vi "Example.vi"() -> ()   [LabVIEW 2024]
uses:
  Users/crogers/GitHub/ME121-25/LabVIEW/SerialVIs/subs/portX.xctl
panel:
  in  "CtrlC":bool
  in  "Send Code":bool
  in  "Code to run":string="import time\n\nfor i in range(10):\n    print(i)\n    time.sleep(1)\n"
  in  "portX":refnum<visa-resource-name>(xcontrol)
  in  "Send it":bool
  in  "Stop Button":bool
  in  "Single line":string="2+2"
  out "reply":string
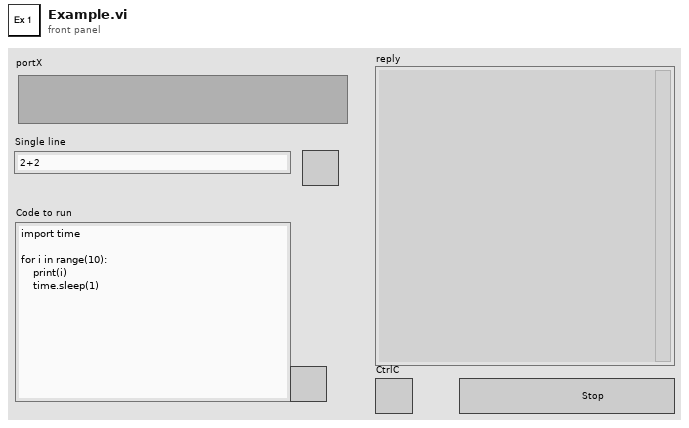
[diagram p1: front panel]
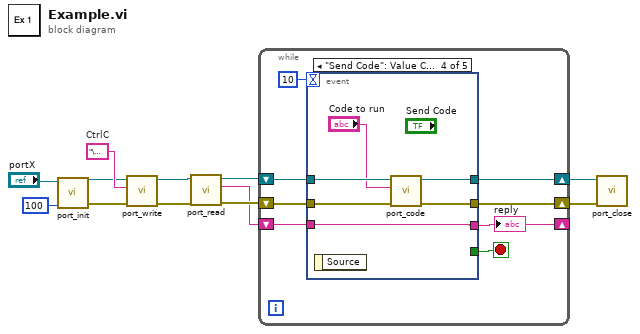
[diagram p0: block diagram]
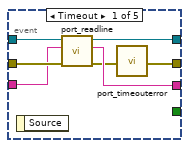
[diagram p2: hidden frame]
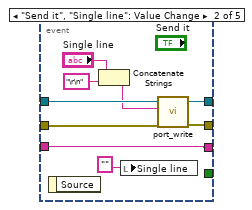
[diagram p3: hidden frame]
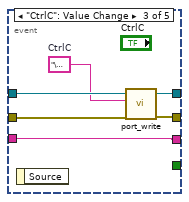
[diagram p4: hidden frame]
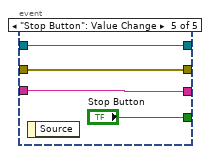
[diagram p5: hidden frame]
diagram:
  w12 = "\u0003"  # CtrlC
  n1 = call <userlib>:"port_init.vi"("Timeout (ms)"=u32 100, "VISA Refnum in"="portX") -> ("error out"=w10:errorcluster, "VISA Refnum out"=w11:refnum<visa-resource-name>)  [unwired: 8 in]
  n2 = call <userlib>:"port_write.vi"("error in (no error)"=w10, "write buffer"=w12, "VISA Refnum in"=w11) -> ("error out"=w6:errorcluster, "VISA Refnum out"=w7:refnum<visa-resource-name>)  [unwired: 7 in]
  n3 = call <userlib>:"port_read.vi"("error in (no error)"=w6, "VISA Refnum in"=w7) -> ("error out"=w5:errorcluster, "reply"=w3:string, "VISA Refnum out"=w4:refnum<visa-resource-name>)  [unwired: 7 in]
  n4 = while {
    shift-right: [w17] -> w8
    shift-left: w4 -> [w20]
    shift-right: [w18] -> w9
    shift-left: w5 -> [w19]
    shift-right: [w14] -> _
    shift-left: w3 -> [w13]
    stop <- w16 stop-if-true
    n5 = event shown="[3] \"Send Code\": Value Change" {
      selector: _ -> [_ _ _ _ _]
      dyn-events: _ -> [_ _ _ _ _]
      timeout: 10 -> [_ _ _ _ _]
      tunnel: w20 -> [w26 w34 w40 w46 w52]
      tunnel: w19 -> [w27 w33 w39 w45 w51]
      tunnel: [w21 w36 w42 w48 w51] -> w18
      tunnel: [w24 w35 w41 w47 w52] -> w17
      tunnel: [_ _ _ _ "Stop Button"] -> w16
      tunnel: [w23 w28 w38 w44 w49] -> w14
      tunnel: w13 -> [w25 w28 w38 w44 w49]
      event Timeout {
        n6 = event-data() -> ()  [unwired: 1 in, 1 out]
        n7 = call <userlib>:"port_readline.vi"("error in (no error)"=w27, "String in"=w25, "VISA Refnum in"=w26) -> ("error out"=w22:errorcluster, "reply"=w23:string, "VISA Refnum out"=w24:refnum<visa-resource-name>)  [unwired: 6 in]
        n8 = call <userlib>:"port_timeouterror.vi"("error in (no error)"=w22) -> ("error out"=w21:errorcluster)  [unwired: 10 in]
      }
      event "Send it", "Single line": Value Change {
        n9 = event-data() -> ()  [unwired: 1 in, 1 out]
        n10 = Concatenate Strings("Single line", "\r\n" ("string")) -> (w31:string)
        n11 = local write "Single line"("" ("string")) -> ()
        n12 = call <userlib>:"port_write.vi"("error in (no error)"=w33, "write buffer"=w31, "VISA Refnum in"=w34) -> ("error out"=w36:errorcluster, "VISA Refnum out"=w35:refnum<visa-resource-name>)  [unwired: 7 in]
      }
      event "CtrlC": Value Change {
        w37 = "\u0003"  # CtrlC
        n13 = event-data() -> ()  [unwired: 1 in, 1 out]
        n14 = call <userlib>:"port_write.vi"("error in (no error)"=w39, "write buffer"=w37, "VISA Refnum in"=w40) -> ("error out"=w42:errorcluster, "VISA Refnum out"=w41:refnum<visa-resource-name>)  [unwired: 7 in]
      }
      event "Send Code": Value Change {
        n15 = event-data() -> ()  [unwired: 1 in, 1 out]
        n16 = call <userlib>:"port_code.vi"("error in (no error)"=w45, "Code to run"="Code to run", "VISA Refnum in"=w46) -> ("error out"=w48:errorcluster, "VISA Refnum out"=w47:refnum<visa-resource-name>)  [unwired: 7 in]
      }
      event "Stop Button": Value Change {
        n17 = event-data() -> ()  [unwired: 1 in, 1 out]
      }
    }
    "reply" <- w14
  }
  n18 = call <userlib>:"port_close.vi"("error in (no error)"=w9, "VISA Refnum in"=w8) -> ()  [unwired: 10 in]
